vi "n get xy pos.vi"(8 "error in (no error)":errorcluster, 9 "y":i16, 10 "x":i16, 11 "n":u16) -> (0 "error out":errorcluster, 1 "y out":i16, 2 "x out":i16)   [LabVIEW 2015, in "SCANalone4x64.lvlib"]
doc: "__declspec(dllimport) void __stdcall n_get_xy_pos(unsigned short n, short *x, short *y);"
uses:
  <userlib>/SCANalone4x64/SCANalone4x64.lvlib
  <userlib>/SCANalone4x64/SCANalone4x64.dll
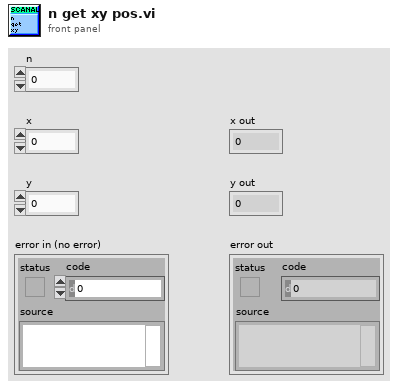
[diagram p1: front panel]
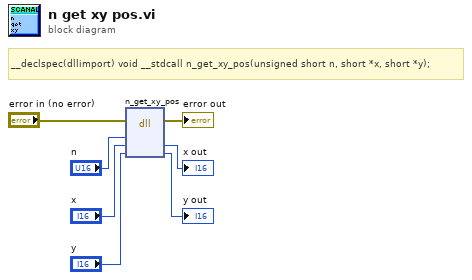
[diagram p0: block diagram]
diagram:
  # "__declspec(dllimport) void __stdcall n_get_xy_pos(unsigned short n, short *x, short *y);"
  n1 = dll-call lib="C:/Program Files/National Instruments/LabVIEW 2015/user.lib/SCANalone4x64/SCANalone4x64.*" fn="n_get_xy_pos"(error in="error in (no error)", "n"="n", "x"="x", "y"="y") -> (error out=→"error out":errorcluster, "x"=→"x out":i16, "y"=→"y out":i16)  [unwired: 4 in, 1 out]
